vi "Start.vi"(8 "error in (no error)":errorcluster, 11 "Task in":refnum<class "Channel.lvclass">) -> (0 "error out":errorcluster, 3 "Task out":refnum<class "Channel.lvclass">)   [LabVIEW 2009, in "MicroDAQ.lvlib" / "Channel.lvclass"]
uses:
  <instrlib>/MicroDAQ/Channel/Channel.lvclass
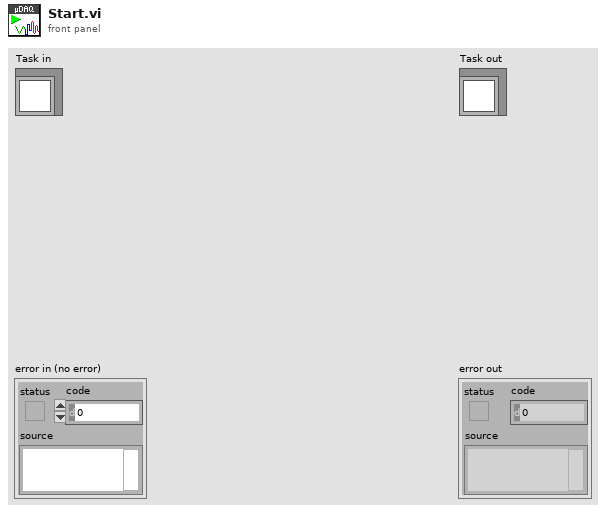
[diagram p1: front panel]
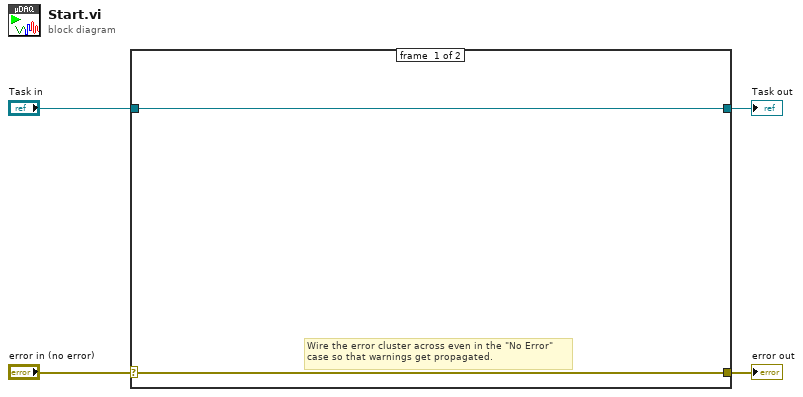
[diagram p0: block diagram]
diagram:
  n1 = case shown="No Error" "error in (no error)" {
    selector: "error in (no error)" -> [w5 w8]
    tunnel: [w5 w8] -> w3
    tunnel: [w6 w7] -> w1
    tunnel: "Task in" -> [w6 w7]
    frame #0 {
      # "Wire the error cluster across even in the \"No Error\"\ncase so that warnings get propagated."
    }
    frame #1 {
    }
  }
  "error out" <- w3
  "Task out" <- w1
